vi "solar_write SubscribeThisQ.vi"(8 "error in (no error)":errorcluster, 10 "Publisher Target":string, 11 "solar in":refnum<class "solar.lvclass">) -> (0 "error out":errorcluster, 3 "solar out":refnum<class "solar.lvclass">)   [LabVIEW 2018, in "solar.lvclass"]
doc: "This subscribes this target's queue to receive telemetry from the destination target whenever the destination target returns telemetry. The messages returned are prefixed with the destination target's name (i.e. 'TARGET:TLM')\nNote: The destination target cannot be this target, this would cause an infinite loop scenario."
uses:
  solar.lvclass
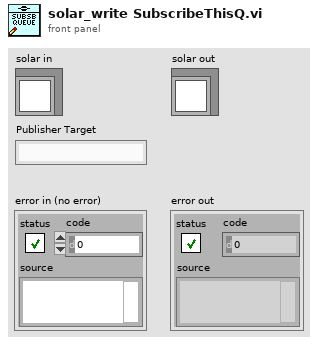
[diagram p1: front panel]
types:
  T1 = typedef "solar_ctl SOLAR Refnum.ctl" = refnum<k1>
  T2 = typedef "solar_ctl SOLAR Global.ctl" = cluster{"Targets":T3[], "AppDir":path, "solar.ini":path, "ConfigsDir":path, "CosmosDir":path, "LogsDir":path, "ExePath":path, "ExeVersion":string, "PartNum":string, "AppSetup":string, "Title":string, "Main.ini":path, "Temp.ini":path, "vSOLAR":string, "Splash.png":string, "SplashWait":i32, "SOLARUE":refnum<user-event>, "VoyagerRefnum":T4, "QTimerRefnum":T5}
  T3 = typedef "solar_ctl Target Global.ctl" = cluster{"Target":string, "Q":refnum<queue>, "UE":refnum<user-event>, "VI":refnum<vi>, "Menu":refnum<k9>, "Data":refnum<data-value>, "Attributes":variant}
  T4 = typedef "solar_voy_ctl Voyager Refnum.ctl" = refnum<k1>
  T5 = typedef "solar_qtimer_ctl Refnum.ctl" = refnum<k1>
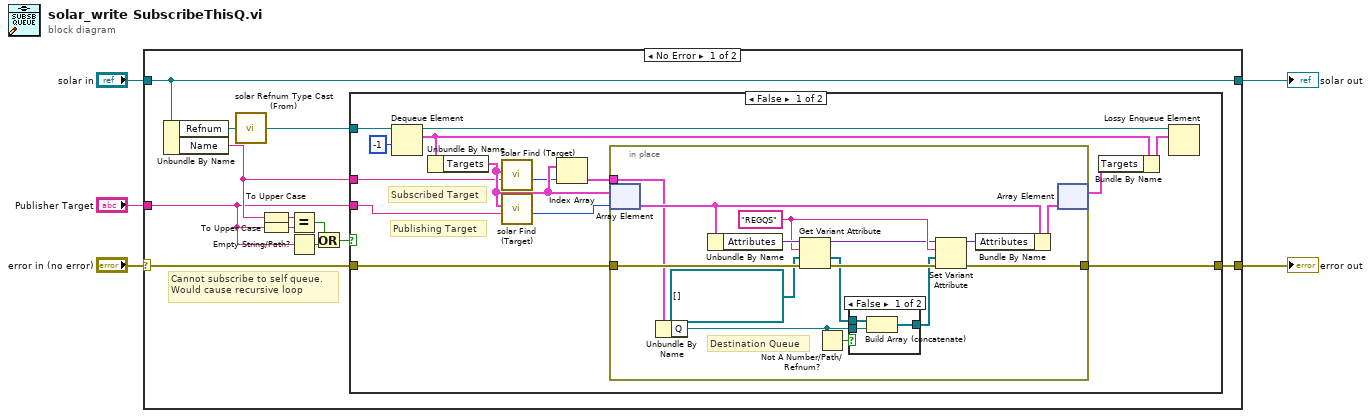
[diagram p0: block diagram]
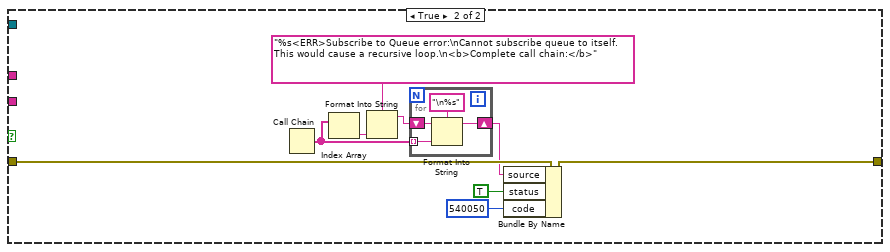
[diagram p3: hidden frame]
diagram:
  n1 = case shown="No Error" "error in (no error)" {
    selector: "error in (no error)" -> [w16 w65]
    tunnel: "solar in" -> [w17 w64]
    tunnel: [w13 w65] -> w2
    tunnel: [w17 w64] -> w1
    tunnel: "Publisher Target" -> [w7 _]
    frame No Error {
      # "Cannot subscribe to self queue.\nWould cause recursive loop"
      n2 = Unbundle By Name(w17) -> ("Refnum"=w15:T1, "Name"=w8:string)
      n3 = call "solar Refnum Type Cast (From).vi"("Refnum"=w15) -> ("SOLAR"=w14:refnum<queue>)
      n4 = To Upper Case(1:w8) -> (0:w9:string)
      n5 = To Upper Case(1:w7) -> (0:w10:string)
      n6 = Equal?(x=w9, y=w10) -> (x = y?=w11:bool)
      n7 = Empty String/Path?(string/path=w7) -> (empty?=w12:bool)
      n8 = Or(x=w11, y=w12) -> (x .or. y?=w6:bool)
      n9 = case shown="False" w6 {
        tunnel: w16 -> [w31 w53]
        tunnel: w14 -> [w30 _]
        tunnel: [w27 w51] -> w13
        tunnel: w8 -> [w19 _]
        tunnel: w7 -> [w18 _]
        frame False {
          # "Publishing Target"
          # "Subscribed Target"
          n10 = Dequeue Element(queue=w30, timeout in ms (-1)=-1) -> (queue out=w29:refnum<queue>, element=w26:T2)  [unwired: 1 in, 2 out]
          n11 = Unbundle By Name(w26) -> ("Targets"=w22:T3[])
          n12 = call "solar Find (Target).vi"("Target"=w19, "Targets"=w22) -> ("Target Index"=w21:i32)  [unwired: 8 in, 1 out]
          n13 = call "solar Find (Target).vi"("Target"=w18, "Targets"=w22) -> ("Target Index"=w24:i32)  [unwired: 8 in, 1 out]
          n14 = Index Array(array=w22, index=w21) -> (element=w20:T3)
          n15 = in-place {
            in-place-border: w31 -> [w43]
            in-place-border: [w42] -> w27
            in-place-border: w20 -> [w32]
            w39 = "REGQS" ("name")
            # "Destination Queue"
            n16 = in-place-array #1(w22, w24) -> (w46:T3)
            n17 = Unbundle By Name(w32) -> ("Q"=w33:refnum<queue>)
            n18 = Unbundle By Name(w46) -> ("Attributes"=w40:variant)
            n19 = Get Variant Attribute(Variant=w40, name=w39, default value (empty Variant)=refnum<queue>[] [] ("RegQs"), error in=w43) -> (duplicate Variant=w37:variant, value=w35:refnum<queue>[], error out=w41:errorcluster)  [unwired: 1 out]
            n20 = Not A Number/Path/Refnum?(number/path/refnum=w33) -> (NaN/Path/Refnum?=w36:bool)
            n21 = case shown="False" w36 {
              tunnel: w35 -> [w49 w50]
              tunnel: [w48 w50] -> w34
              tunnel: w33 -> [w47 _]
              frame False {
                n22 = Build Array (concatenate)(w49, w47) -> (w48:refnum<queue>[])
              }
              frame True {
              }
            }
            n23 = Set Variant Attribute(Variant=w37, name=w39, value=w34, error in=w41) -> (Variant out=w44:variant, error out=w42:errorcluster)  [unwired: 1 out]
            n24 = Bundle By Name(cluster=w46, "Attributes"=w44) -> (w45:T3)
            n25 = in-place-array #1(w45) -> (w23:T3[])  [unwired: 1 out]
          }
          n26 = Bundle By Name(cluster=w26, "Targets"=w23) -> (w25:T2)
          n27 = Lossy Enqueue Element(queue=w29, element=w25) -> ()  [unwired: 1 in, 4 out]
        }
        frame True {
          n28 = Call Chain() -> (call chain=w54:string[])
          n29 = Index Array(array=w54) -> (element=w56:string)  [unwired: 1 in]
          n30 = Format Into String(format string="%s<ERR>Subscribe to Queue error:\nCannot subscribe queue to itself. This would cause a recursive loop.\n<b>Complete call chain:</b>", w56) -> (resulting string=w55:string)  [unwired: 2 in, 1 out]
          n31 = for {
            tunnel: w54 -> [w63] mode=indexing
            shift-right: [w62] -> w52
            shift-left: w55 -> [w61]
            n32 = Format Into String(format string="\n%s", initial string=w61, w63) -> (resulting string=w62:string)  [unwired: 1 in, 1 out]
          }
          n33 = Bundle By Name(cluster=w53, "source"=w52, "status"=TRUE, "code"=540050 ("Code")) -> (w51:errorcluster)
        }
      }
    }
    frame Error {
    }
  }
  "error out" <- w2
  "solar out" <- w1
